vi "Apply.vi"(8 "Error In":errorcluster, 11 "Acquire Continuous Waveform CFG":refnum<class "Continuous Waveform Acq CFG.lvclass">) -> (0 "Error Out":errorcluster, 3 "Acquire Continuous Waveform CFG out":refnum<class "Continuous Waveform Acq CFG.lvclass">)   [LabVIEW 2023, in "RIGOL DS1054.lvlib" / "Continuous Waveform Acq CFG.lvclass"]
uses:
  Continuous Waveform Acq CFG.lvclass
  Scope VISA/Configuration/Scope VISA CFG.lvclass
  <instrlib>/RIGOL DS1000 Series/RIGOL DS1000 Series.lvlib
  D:/git/HAL/Scope VISA/Configuration/Scope VISA CFG.lvclass
  D:/git/HAL/Scope Base/Configuration/Scope Base CFG.lvclass
  D:/git/HAL/Configuration Base/Configuration Base.lvclass
  D:/git/HAL/Interfaces/IConfigure/IConfigure.lvclass
  D:/git/HAL/Devices/Rigol DS1054/Configurations/Acquire Continuous Waveform/Continuous Waveform Acq CFG.lvclass
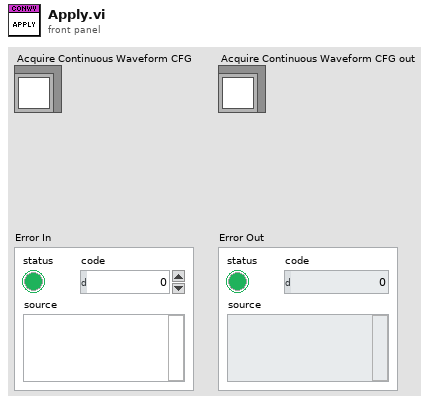
[diagram p1: front panel]
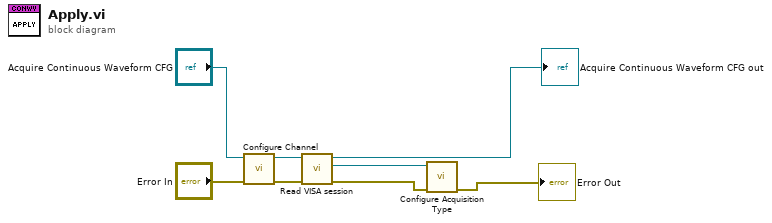
[diagram p0: block diagram]
diagram:
  n1 = call-dynamic "Configure Channel.vi"("error in"="Error In", "Continuous Waveforn Acq CFG in"="Acquire Continuous Waveform CFG") -> ("error out"=w7:errorcluster, "Continuous Waveforn Acq CFG out"=w5:refnum<class "Continuous Waveform Acq CFG.lvclass">)  [unwired: 8 in]
  n2 = call "Read VISA session.vi"("error in (no error)"=w7, "Scope VISA CFG in"=w5) -> ("error out"=w3:errorcluster, "VISA session"=w2:refnum<visa-resource-name>, "Scope VISA CFG out"=→"Acquire Continuous Waveform CFG out":refnum<class "Continuous Waveform Acq CFG.lvclass">)  [unwired: 7 in]
  n3 = call <instrlib>:"Configure Acquisition Type.vi"("error in (no error)"=w3, "VISA resource name"=w2) -> ("error out"=→"Error Out":errorcluster)  [unwired: 8 in, 1 out]
